vi "Typ params.vi"(11 "Analogowe":waveform(dbl)[](array[waveform])) -> (0 "dt":dbl, 1 "Rozm":i32, 2 "Nazwy":string[](array[string]), 3 "L. Kan":i32)   [LabVIEW 2014]
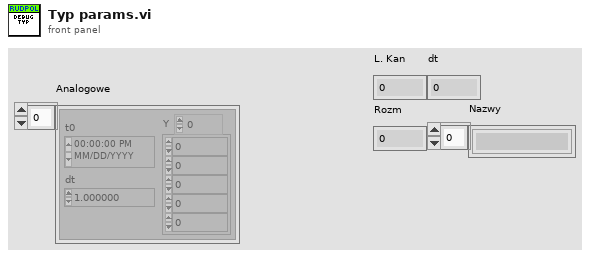
[diagram p1: front panel]
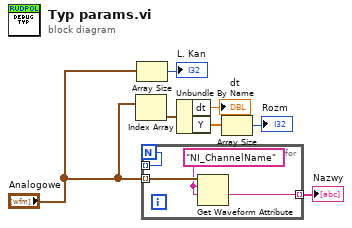
[diagram p0: block diagram]
diagram:
  n1 = Index Array(array="Analogowe") -> (element=w5:waveform(dbl))  [unwired: 1 in]
  n2 = Array Size(array="Analogowe") -> (size(s)=→"L. Kan":i32)
  n3 = for {
    N -> [w8]
    tunnel: "Analogowe" -> [w11] mode=indexing
    tunnel: [w9] -> w1 mode=indexing
    tunnel: [w8] -> _ mode=indexing
    w10 = "NI_ChannelName" ("name")
    n4 = Get Waveform Attribute(5:w10, 6:w10, 7:w11) -> (1:w9:string)  [unwired: 1 in, 3 out]
  }
  "Nazwy" <- w1
  n5 = Unbundle By Name(w5) -> ("dt"=→"dt":dbl, "Y"=w7:dbl[])
  n6 = Array Size(array=w7) -> (size(s)=→"Rozm":i32)
